vi "Actor API Type.vi"(11 "Test 1 in":refnum<class "Test 1.lvclass">) -> (2 "Actor API Type":refnum<class "Actor API.lvclass">)   [LabVIEW 2020, in "Scratchpad.lvlib" / "Test 1.lvlib" / "Test 1.lvclass"]
uses:
  Test 1.lvclass
  Test 1 API/Test 1 API.lvclass
  Artifex/Actor Proxy/Actor API.lvclass
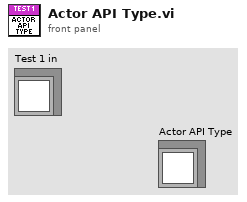
[diagram p1: front panel]
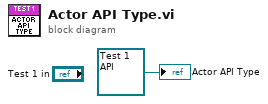
[diagram p0: block diagram]
diagram:
  "Actor API Type" <- refnum<class "Test 1 API.lvclass"> refnum ("Scratchpad.lvlib:Test 1.lvlib:Test 1 API.lvclass")
